vi "Test V Mode Sens.vi"(8 "error in (no error)":errorcluster, 11 "SR7270 Drivers in":refnum<class "SR7270 Drivers.lvclass">) -> (0 "error out":errorcluster, 3 "SR7270 Drivers out":refnum<class "SR7270 Drivers.lvclass">)   [LabVIEW 2016, in "SR7270 Drivers.lvclass"]
uses:
  SR7270 Drivers.lvclass
  Typedefs/SEN-IMODE0--enum.ctl
  SR7270 Drivers.lvclass/SR7270 Drivers.ctl
  <vilib>/addons/_JKI Toolkits/Caraya/classes/Assert/Assert.lvclass
  <vilib>/addons/_JKI Toolkits/Caraya/classes/Test/Test.lvclass
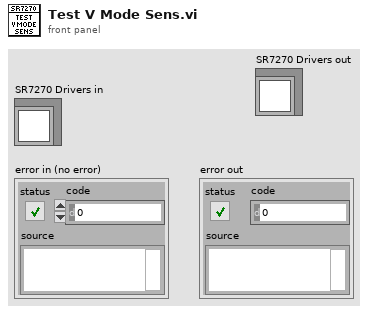
[diagram p1: front panel]
types:
  T1 = typedef "SR7270 Drivers.lvclass/SEN-IMODE0--enum.ctl" = enum16{"2 nV", "5 nV", "10 nV", "20 nV", "50 nV", "100 nV", "200 nV", "500 nV", "1 µV", "2 µV", "5 µV", "10 µV", "20 µV", "50 µV", "100 µV", "200 µV", "500 µV", "1 mV", "2 mV", "5 mV", "10 mV", "20 mV", "50 mV", "100 mV", "200 mV", "500 mV", "1 V"}
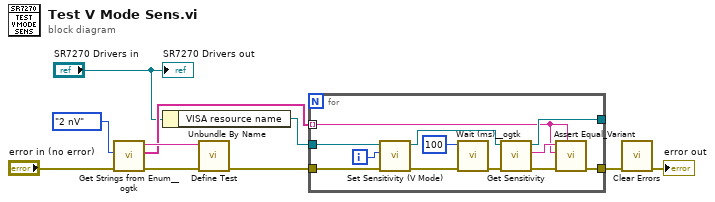
[diagram p0: block diagram]
diagram:
  n1 = call <userlib>:"Get Strings from Enum__ogtk.vi"("error in (no error)"="error in (no error)", "Enum"=SEN-IMODE0--enum."2 nV" ("Sensitivity IMODE0")) -> ("error out"=w3:errorcluster, "Enum Strings"=w6:string[], "Enum Name"=w7:string)  [unwired: 6 in, 1 out]
  n2 = Unbundle By Name("SR7270 Drivers in") -> ("VISA resource name"=w2:refnum<visa-resource-name>)
  n3 = call <vilib>:"Define Test.vi"("error in (no error)"=w3, "Label (VI Title)"=w7) -> ("error out"=w10:errorcluster)  [unwired: 9 in]
  n4 = for {
    tunnel: w2 -> [w21]
    tunnel: w10 -> [w13]
    tunnel: [w19] -> w9
    tunnel: [w18] -> _
    tunnel: w6 -> [w11] mode=indexing
    i -> [w12]
    n5 = call "Set Sensitivity (V Mode).vi"("error in (no error)"=w13, "Sensitivity IMODE0"=w12, "VISA resource name"=w21) -> ("error out"=w15:errorcluster, "VISA resource name out"=w22:refnum<visa-resource-name>)  [unwired: 7 in]
    n6 = call <userlib>:"Wait (ms)__ogtk.vi"("error in (no error)"=w15, "milliseconds to wait"=u32 100) -> ("error out"=w17:errorcluster)  [unwired: 8 in, 1 out]
    n7 = call "Get Sensitivity.vi"("error in (no error)"=w17, "VISA resource name"=w22) -> ("error out"=w20:errorcluster, "Sensitivty"=w14:string, "VISA resource name out"=w18:refnum<visa-resource-name>)  [unwired: 6 in, 1 out]
    n8 = call <vilib>:"Assert Equal_Variant.vi"("Label"=w11, "error in (no error)"=w20, "Y"=w11, "X"=w14) -> ("error out"=w19:errorcluster)  [unwired: 7 in]
  }
  n9 = call <vilib>:"Clear Errors.vi"("error in (no error)"=w9) -> ("error out"=→"error out":errorcluster)  [unwired: 5 in, 1 out]
  "SR7270 Drivers out" <- "SR7270 Drivers in"
